vi "Log.vi"(7 "Level":T1(ring), 8 "error in (no error)":errorcluster, 9 "error":errorcluster, 10 "Message":string, 11 "Logger in":refnum<class "Logger.lvclass">) -> (0 "error out":errorcluster, 3 "Logger out":refnum<class "Logger.lvclass">)   [LabVIEW 2017, in "Error Log.lvlib" / "Logger.lvclass"]
doc: "Creates a ``Record`` with the specified <b>Level</b>, <b>Message</b> and <b>error</b>, and passes it to the registered ``Handlers``."
uses:
  Logger.lvclass
  Logger.lvclass/Logger.ctl
  Get Handlers.vi
  Get Display Format.vi
  Record.Error/Record.Error.lvclass
  \\192.168.1.40\Neosoft/Partage/Dossiers Personnels/BRO/DevTools_BR/wc/ErrorLog/src/Record/Record.lvclass
  Handler/Handler.lvclass
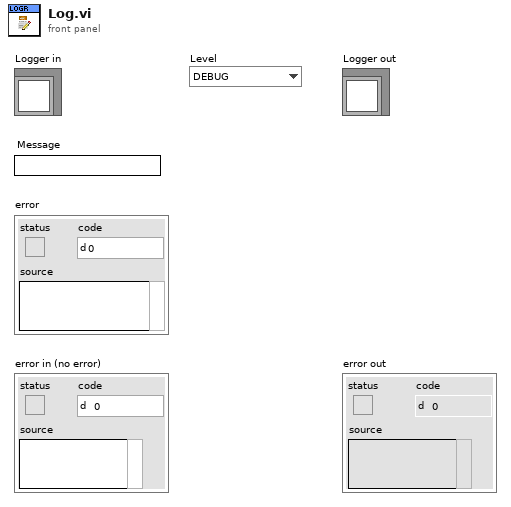
[diagram p1: front panel]
types:
  T1 = enum16{"DEBUG", "INFO", "WARNING", "ERROR", "CRITICAL"}
  T2 = typedef "Error Log.lvlib/Display Format.ctl" = enum16{"PlainText", "PlainText.INI", "XML", "JSON"}
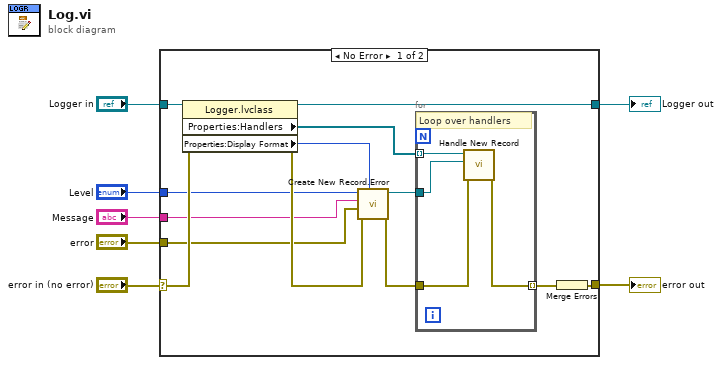
[diagram p0: block diagram]
diagram:
  n1 = case shown="No Error" "error in (no error)" {
    selector: "error in (no error)" -> [w20 w26]
    tunnel: [w13 w26] -> w6
    tunnel: [w11 w25] -> w4
    tunnel: "Logger in" -> [w15 w25]
    tunnel: "Level" -> [w18 _]
    tunnel: "Message" -> [w17 _]
    tunnel: "error" -> [w16 _]
    frame No Error {
      n2 = property class="Logger.lvclass"(reference=w15, error in=w20) -> (reference out=w11:refnum<class "Logger.lvclass">, error out=w19:errorcluster, "Properties:Handlers"=w10:refnum<class "Handler.lvclass">[], "Properties:Display Format"=w8:T2)
      n3 = call "Create New Record.Error.vi"("Display Format"=w8, "error in (no error)"=w19, "Error"=w16, "Message"=w17, "Level"=w18) -> ("error out"=w9:errorcluster, "Record.Error out"=w12:refnum<class "Record.Error.lvclass">)  [unwired: 5 in]
      n4 = for {
        tunnel: w10 -> [w24] mode=indexing
        tunnel: w9 -> [w22]
        tunnel: [w21] -> w14 mode=indexing
        tunnel: w12 -> [w23]
        # "Loop over handlers"
        n5 = call "Handle New Record.vi"("error in (no error)"=w22, "New Record"=w23, "Handler in"=w24) -> ("error out"=w21:errorcluster)  [unwired: 7 in, 1 out]
      }
      n6 = Merge Errors(w14) -> (w13:errorcluster)
    }
    frame Error {
    }
  }
  "error out" <- w6
  "Logger out" <- w4
